vi "Phsae_shift_test(4).vi"() -> ()   [LabVIEW 2017]
uses:
  <vilib>/Analysis/3filter.llb/Filter Passband Type.ctl
  <vilib>/Analysis/3filter.llb/FIR Windowed Filter (DBL).vi
  <vilib>/Analysis/NI_AALBase.lvlib
  <vilib>/Analysis/NI_AALPro.lvlib
panel:
  out "S3 signal":waveform(dbl)(graph)
  out "S2 signal":waveform(dbl)(graph)
  out "S1 signal":waveform(dbl)(graph)
  out "S0 signal":waveform(dbl)(graph)
  out "doppler frequency %":dbl
  in  "Carrier Dopphler On":bool
  in  "DpF":dbl=10000.0
  in  "signal Dopphler On":bool
  out "S0 signal(LPF)":waveform(dbl)(graph)
  out "S1 signal(LPF)":waveform(dbl)(graph)
  out "S2 signal(LPF)":waveform(dbl)(graph)
  out "S3 signal(LPF)":waveform(dbl)(graph)
  out "SUM signal":waveform(dbl)(graph)
  out "최대값":dbl
  in  "Delay time.A.1(sec)":dbl=0.5
  in  "Sampling frequency(Hz)":dbl=3000000.0
  in  "Pulse length(sec)":dbl=0.5
  in  "Amplitude(Vpeak)":dbl=1.0
  in  "Frequency(Hz)":dbl=614000.0
  in  "Carrier Frequency(Hz)":dbl=574000.0
  in  "S0 Phsae":dbl=90.0
  in  "S1 Phsae":dbl=-90.0
  in  "S2 Phsae":dbl=-180.0
  in  "S3 Phsae":dbl=-270.0
  in  "S0 Carrier Phsae":dbl=90.0
  in  "S1 Carrier Phsae":dbl=-90.0
  in  "S2 Carrier Phsae":dbl=-180.0
  in  "S3 Carrier Phsae":dbl=-270.0
  out "S0 FFT":waveform(dbl)(graph)
  out "S1 FFT":waveform(dbl)(graph)
  out "S2 FFT":waveform(dbl)(graph)
  out "S3 FFT":waveform(dbl)(graph)
  out "크기":i32
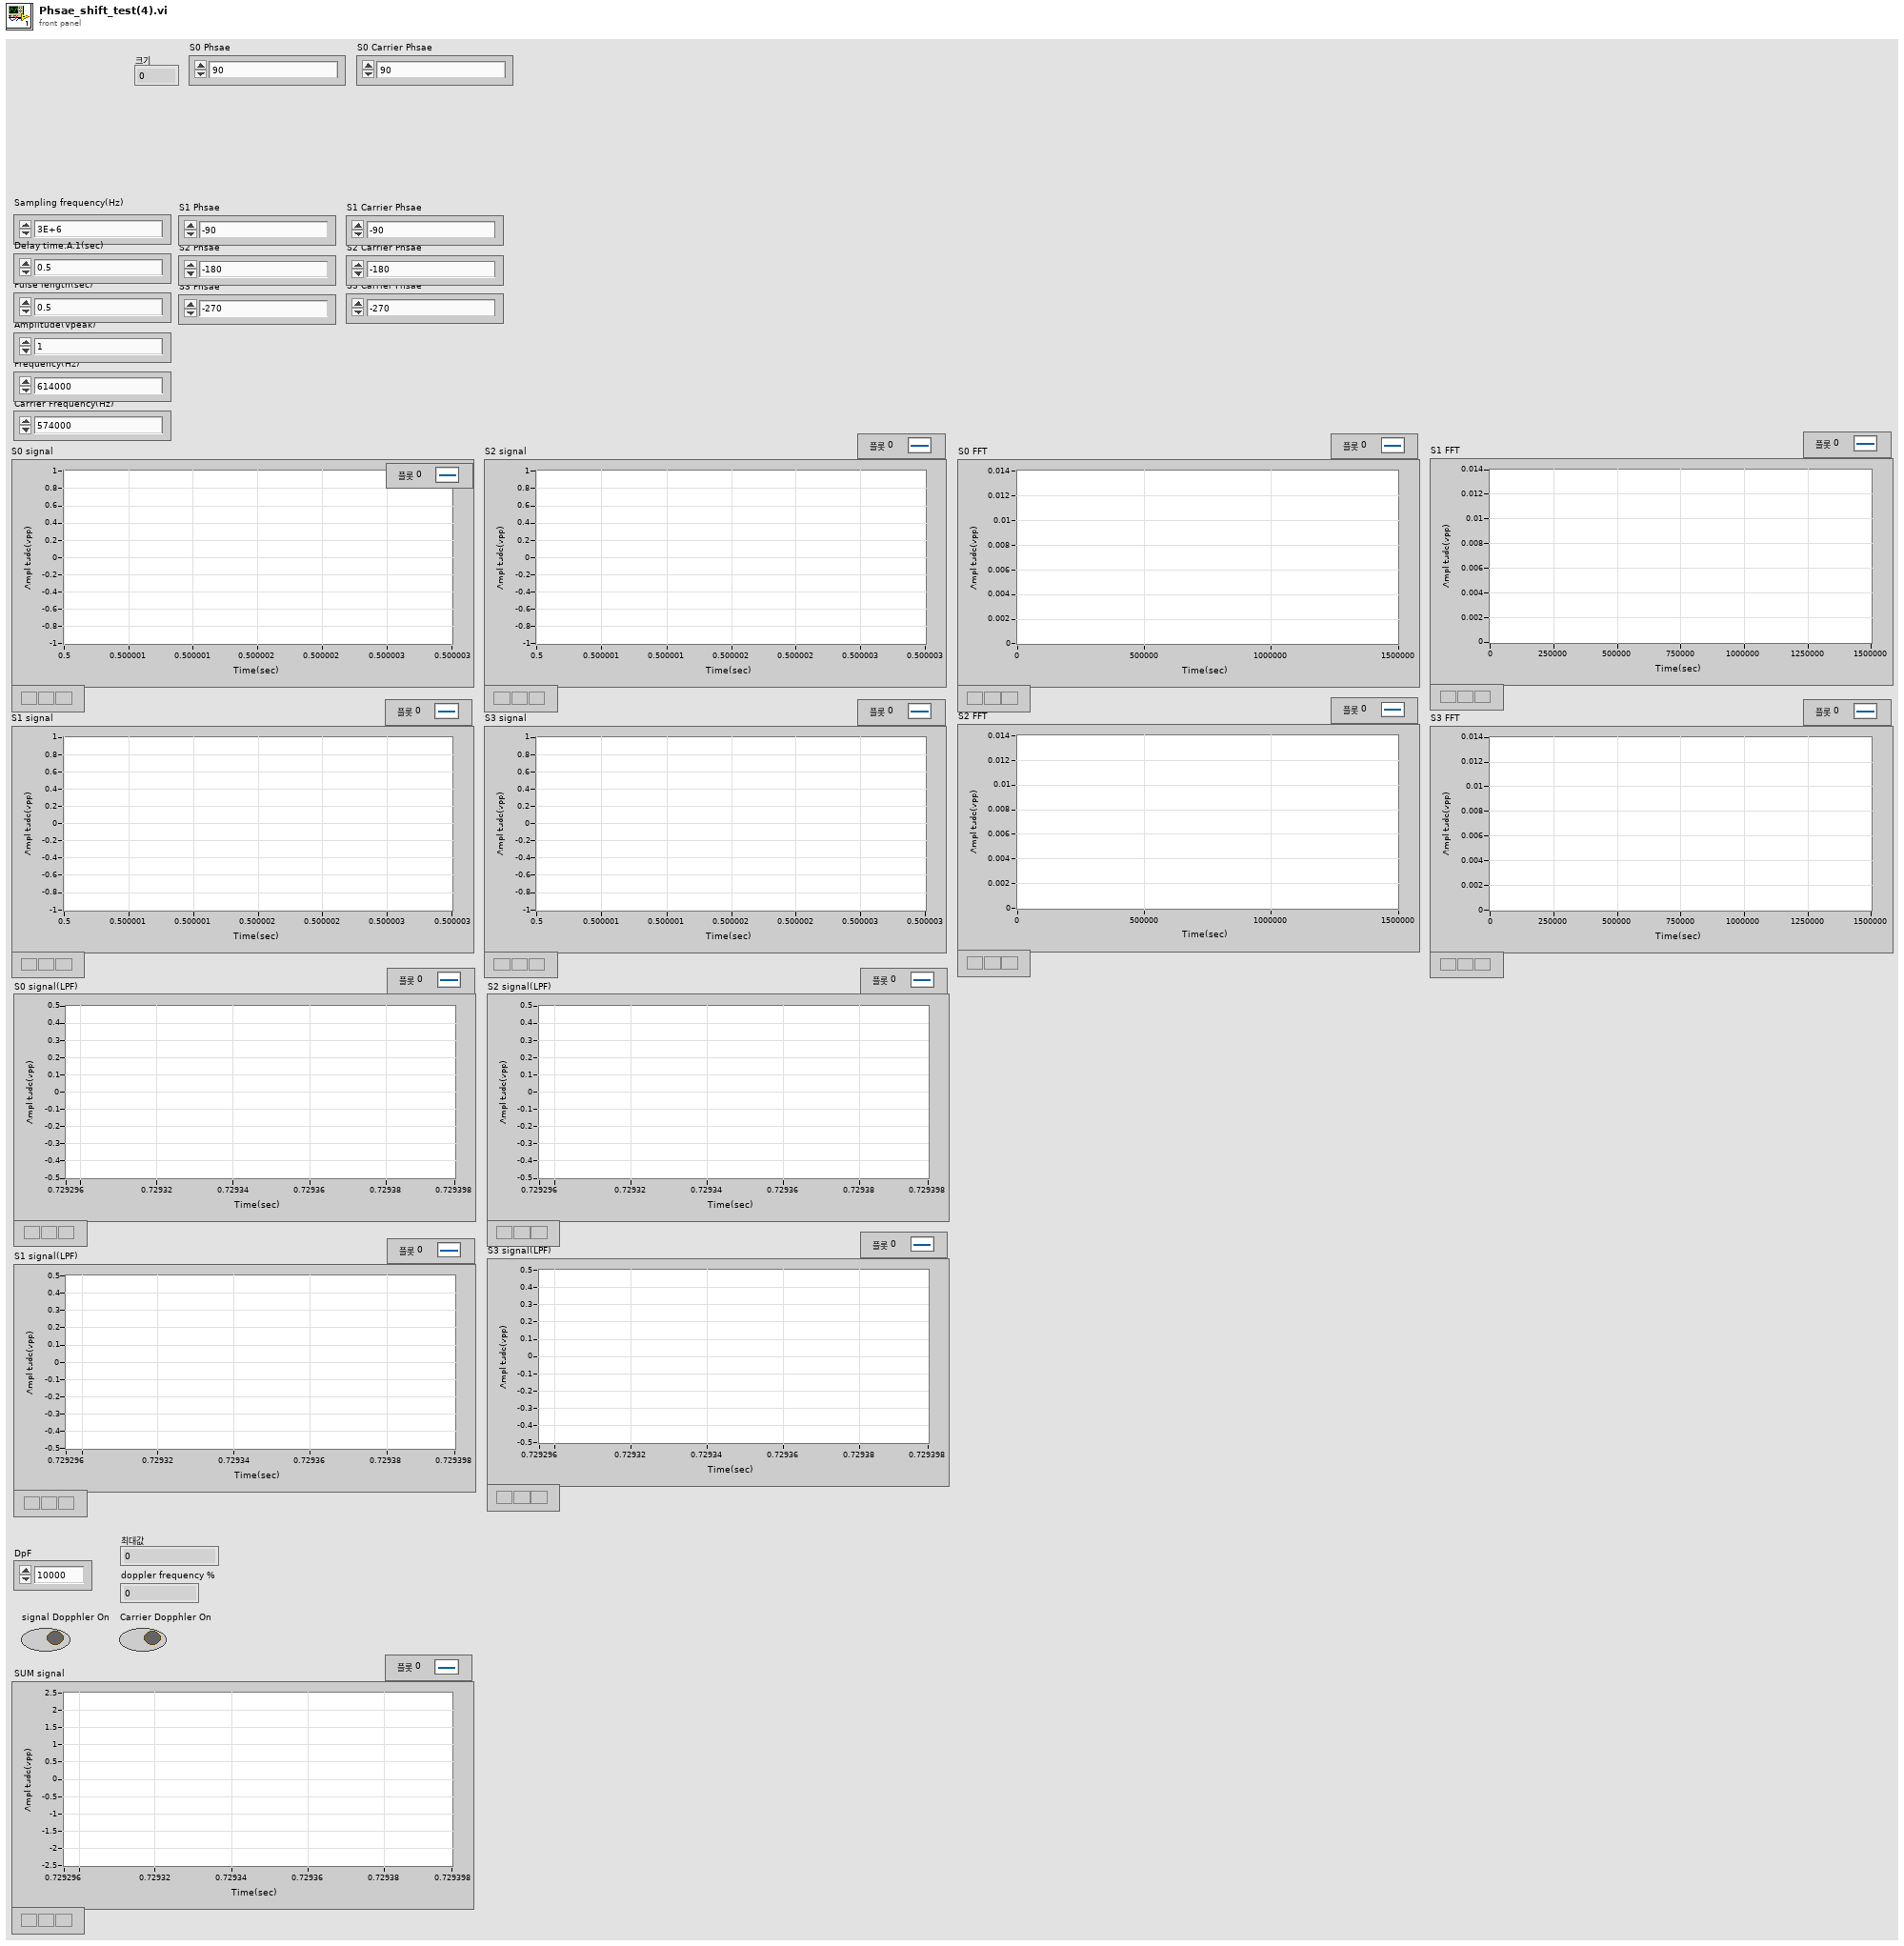
[diagram p1: front panel]
types:
  T1 = typedef "NI_AALBase.lvlib/Filter Passband Type.ctl" = enum32{"Lowpass", "Highpass", "Bandpass", "Bandstop"}
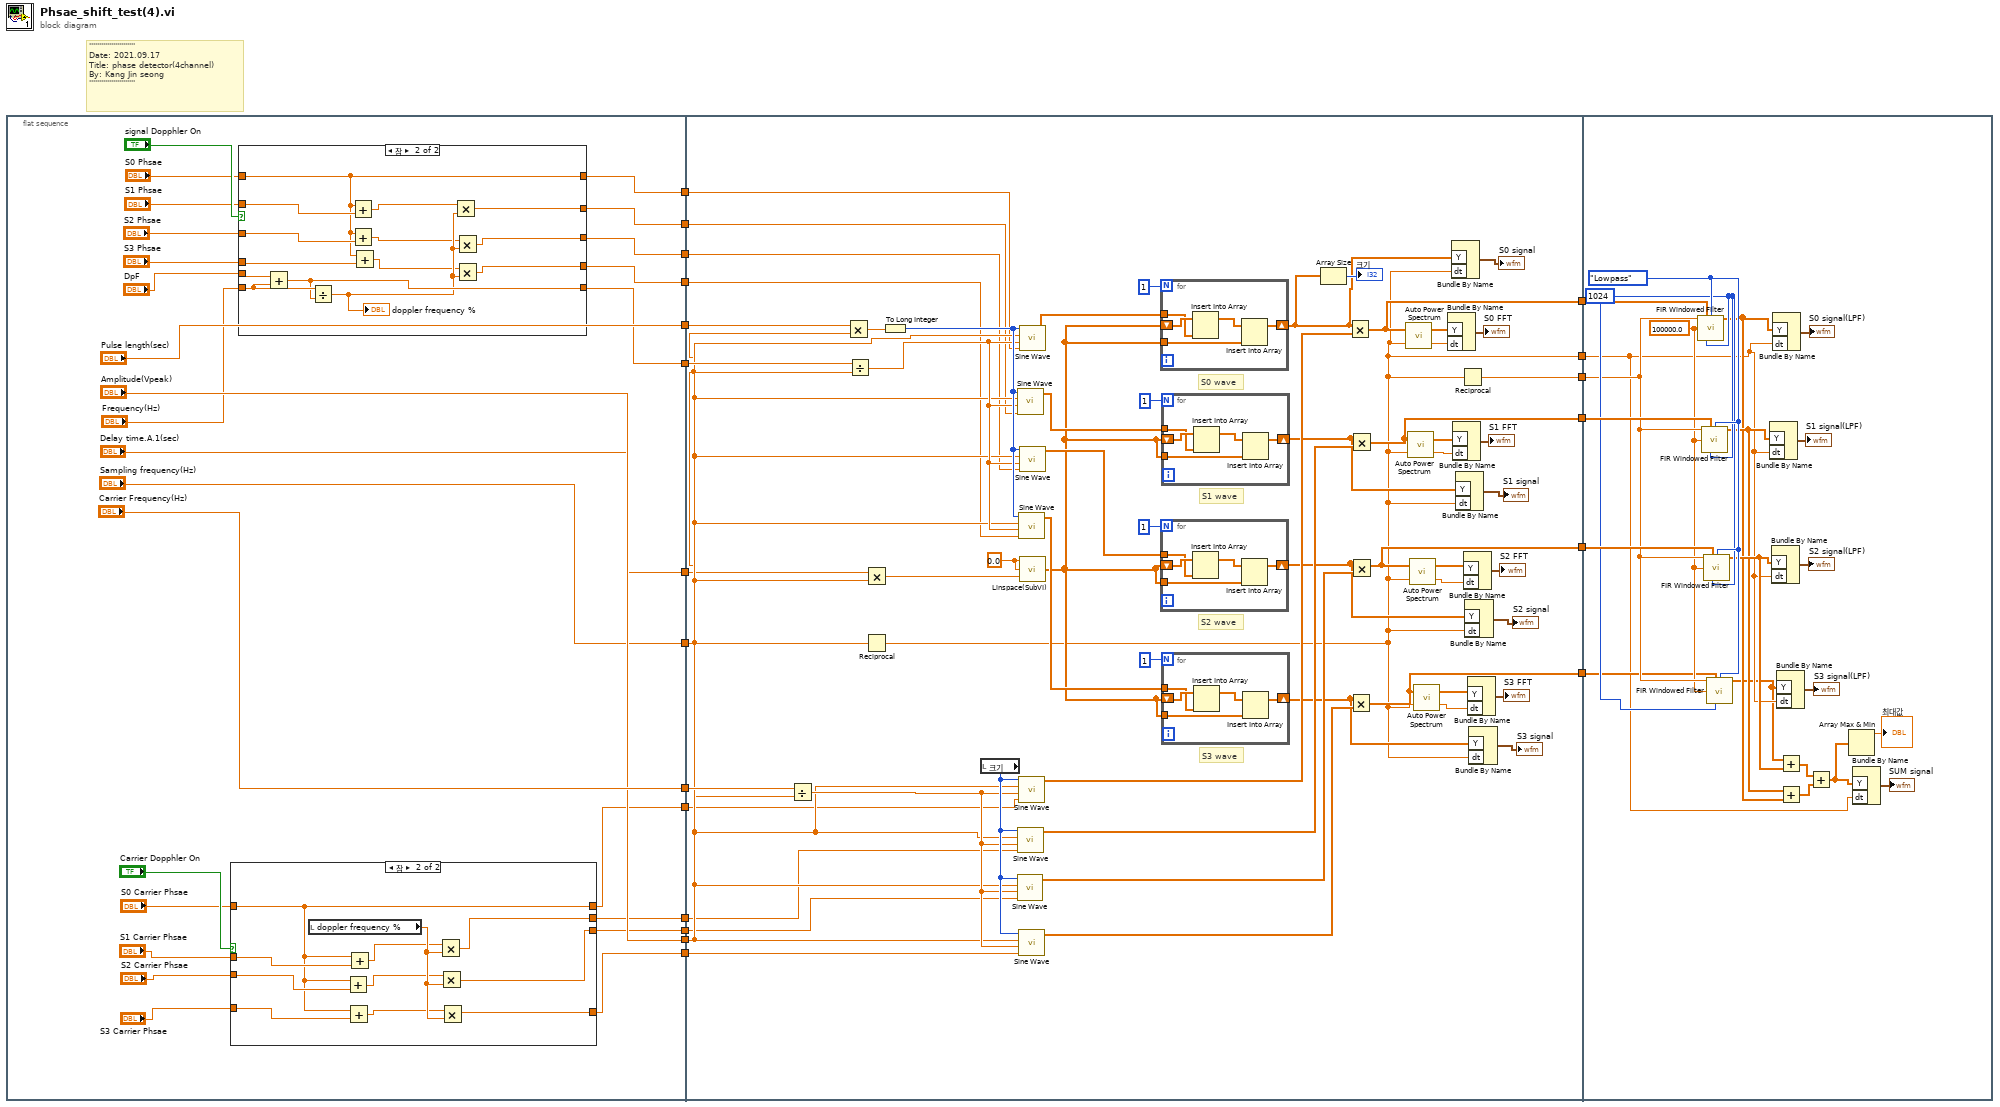
[diagram p0: block diagram]
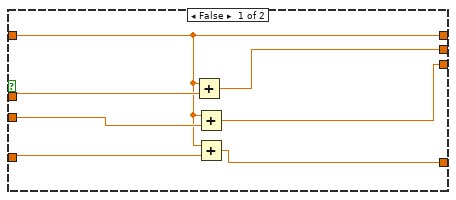
[diagram p2: hidden frame]
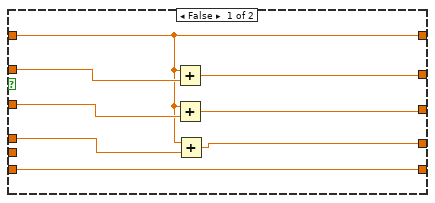
[diagram p3: hidden frame]
diagram:
  # "'''''''''''''''''''''''\nDate: 2021.09.17\nTitle: phase detector(4channel)\nBy: Kang Jin seong\n'''''''''''''''''''''''"
  n1 = flat-sequence {
    tunnel: ["Carrier Frequency(Hz)"] -> w14
    tunnel: [w32] -> w13
    tunnel: ["Amplitude(Vpeak)"] -> w12
    tunnel: ["Pulse length(sec)"] -> w11
    tunnel: ["Sampling frequency(Hz)"] -> w10
    tunnel: ["Delay time.A.1(sec)"] -> w9
    tunnel: [w37] -> w8
    tunnel: [w36] -> w7
    tunnel: [w35] -> w6
    tunnel: [w34] -> w5
    tunnel: [w25] -> w4
    tunnel: [w24] -> w3
    tunnel: [w23] -> w2
    tunnel: [w22] -> w1
    tunnel: [w121] -> w20
    tunnel: [w102] -> w19
    tunnel: [w99] -> w18
    tunnel: [w87] -> w17
    tunnel: [w91] -> w16
    tunnel: [w95] -> w15
    tunnel: w14 -> [w117]
    tunnel: w13 -> [w116]
    tunnel: w12 -> [w115]
    tunnel: w11 -> [w114]
    tunnel: w10 -> [w113]
    tunnel: w9 -> [w112]
    tunnel: w8 -> [w111]
    tunnel: w7 -> [w110]
    tunnel: w6 -> [w109]
    tunnel: w5 -> [w108]
    tunnel: w4 -> [w107]
    tunnel: w3 -> [w106]
    tunnel: w2 -> [w105]
    tunnel: w1 -> [w104]
    tunnel: w15 -> [w182]
    tunnel: w16 -> [w187]
    tunnel: w17 -> [w175]
    tunnel: w18 -> [w188]
    tunnel: w19 -> [w189]
    tunnel: w20 -> [w184]
    frame #0 {
      n2 = case shown="참" "Carrier Dopphler On" {
        tunnel: "S0 Carrier Phsae" -> [w49 w56]
        tunnel: "S1 Carrier Phsae" -> [w53 w60]
        tunnel: "S2 Carrier Phsae" -> [w51 w58]
        tunnel: "S3 Carrier Phsae" -> [w48 w55]
        tunnel: [w49 w56] -> w25
        tunnel: [w52 w63] -> w24
        tunnel: [w50 w62] -> w23
        tunnel: [w47 w61] -> w22
        frame False {
          n3 = Add(x=w49, y=w53) -> (x+y=w52:dbl)
          n4 = Add(x=w49, y=w51) -> (x+y=w50:dbl)
          n5 = Add(x=w49, y=w48) -> (x+y=w47:dbl)
        }
        frame True {
          n6 = local read "doppler frequency %"() -> (w64:dbl)
          n7 = Add(x=w56, y=w58) -> (x+y=w57:dbl)
          n8 = Add(x=w56, y=w55) -> (x+y=w54:dbl)
          n9 = Add(x=w56, y=w60) -> (x+y=w59:dbl)
          n10 = Multiply(x=w59, y=w64) -> (x*y=w63:dbl)
          n11 = Multiply(x=w57, y=w64) -> (x*y=w62:dbl)
          n12 = Multiply(x=w54, y=w64) -> (x*y=w61:dbl)
        }
      }
      n13 = case shown="참" "signal Dopphler On" {
        tunnel: "S0 Phsae" -> [w67 w75]
        tunnel: "S1 Phsae" -> [w71 w79]
        tunnel: "S2 Phsae" -> [w68 w77]
        tunnel: "S3 Phsae" -> [w66 w74]
        tunnel: [w67 w75] -> w37
        tunnel: [w70 w84] -> w36
        tunnel: [w69 w83] -> w35
        tunnel: [w65 w82] -> w34
        tunnel: "Frequency(Hz)" -> [w72 w85]
        tunnel: [w72 w81] -> w32
        tunnel: "DpF" -> [_ w86]
        frame False {
          n14 = Add(x=w67, y=w71) -> (x+y=w70:dbl)
          n15 = Add(x=w67, y=w68) -> (x+y=w69:dbl)
          n16 = Add(x=w67, y=w66) -> (x+y=w65:dbl)
        }
        frame True {
          n17 = Add(x=w86, y=w85) -> (x+y=w81:dbl)
          n18 = Divide(x=w85, y=w81) -> (x/y=w80:dbl)
          "doppler frequency %" <- w80
          n19 = Add(x=w75, y=w79) -> (x+y=w78:dbl)
          n20 = Add(x=w75, y=w77) -> (x+y=w76:dbl)
          n21 = Add(x=w75, y=w74) -> (x+y=w73:dbl)
          n22 = Multiply(x=w78, y=w80) -> (x*y=w84:dbl)
          n23 = Multiply(x=w76, y=w80) -> (x*y=w83:dbl)
          n24 = Multiply(x=w73, y=w80) -> (x*y=w82:dbl)
        }
      }
    }
    frame #1 {
      w144 = 0.0 ("Start")
      # "S3 wave"
      # "S2 wave"
      # "S1 wave"
      # "S0 wave"
      n25 = Divide(x=w117, y=w113) -> (x/y=w132:dbl)
      n26 = Multiply(x=w114, y=w113) -> (x*y=w147:dbl)
      n27 = Divide(x=w116, y=w113) -> (x/y=w145:dbl)
      n28 = Multiply(x=w112, y=w113) -> (x*y=w143:dbl)
      n29 = Reciprocal(x=w113) -> (1/x=w87:dbl)
      n30 = To Long Integer(number=w147) -> (32bit integer=w146:i32)
      n31 = local read "크기"() -> (w133:i32)
      n32 = call <vilib>:"Sine Wave.vi"("samples"=w133, "amplitude"=w115, "frequency"=w132, "phase in"=w105) -> ("sine wave"=w128:dbl[])  [unwired: 1 in, 2 out]
      n33 = call <vilib>:"Sine Wave.vi"("samples"=w146, "amplitude"=w115, "frequency"=w145, "phase in"=w110) -> ("sine wave"=w139:dbl[])  [unwired: 1 in, 2 out]
      n34 = call <vilib>:"Sine Wave.vi"("samples"=w133, "amplitude"=w115, "frequency"=w132, "phase in"=w106) -> ("sine wave"=w129:dbl[])  [unwired: 1 in, 2 out]
      n35 = call <vilib>:"Sine Wave.vi"("samples"=w146, "amplitude"=w115, "frequency"=w145, "phase in"=w108) -> ("sine wave"=w135:dbl[])  [unwired: 1 in, 2 out]
      n36 = call <vilib>:"Sine Wave.vi"("samples"=w133, "amplitude"=w115, "frequency"=w132, "phase in"=w107) -> ("sine wave"=w131:dbl[])  [unwired: 1 in, 2 out]
      n37 = call <vilib>:"Sine Wave.vi"("samples"=w133, "amplitude"=w115, "frequency"=w132, "phase in"=w104) -> ("sine wave"=w127:dbl[])  [unwired: 1 in, 2 out]
      n38 = call <vilib>:"Sine Wave.vi"("samples"=w146, "amplitude"=w115, "frequency"=w145, "phase in"=w111) -> ("sine wave"=w141:dbl[])  [unwired: 1 in, 2 out]
      n39 = call <vilib>:"Sine Wave.vi"("samples"=w146, "amplitude"=w115, "frequency"=w145, "phase in"=w109) -> ("sine wave"=w137:dbl[])  [unwired: 1 in, 2 out]
      n40 = call "Linspace(SubVI).vi"("NumElements"=w143, "End"=w144, "Start"=w144) -> ("Array"=w134:dbl[])
      n41 = for {
        N: 1 -> [_]
        shift-right: [w163] -> w93
        shift-left: w134 -> [w167]
        tunnel: w141 -> [w166]
        tunnel: w134 -> [w164]
        n42 = Insert Into Array(array=w167, new element=w166) -> (w165:dbl[])  [unwired: 1 in]
        n43 = Insert Into Array(array=w165, new element=w164) -> (w163:dbl[])  [unwired: 1 in]
      }
      n44 = for {
        N: 1 -> [_]
        shift-right: [w153] -> w90
        shift-left: w134 -> [w157]
        tunnel: w137 -> [w156]
        tunnel: w134 -> [w154]
        n45 = Insert Into Array(array=w157, new element=w156) -> (w155:dbl[])  [unwired: 1 in]
        n46 = Insert Into Array(array=w155, new element=w154) -> (w153:dbl[])  [unwired: 1 in]
      }
      n47 = for {
        N: 1 -> [_]
        shift-right: [w158] -> w92
        shift-left: w134 -> [w162]
        tunnel: w139 -> [w161]
        tunnel: w134 -> [w159]
        n48 = Insert Into Array(array=w162, new element=w161) -> (w160:dbl[])  [unwired: 1 in]
        n49 = Insert Into Array(array=w160, new element=w159) -> (w158:dbl[])  [unwired: 1 in]
      }
      n50 = for {
        N: 1 -> [_]
        shift-right: [w148] -> w89
        shift-left: w134 -> [w152]
        tunnel: w135 -> [w151]
        tunnel: w134 -> [w149]
        n51 = Insert Into Array(array=w152, new element=w151) -> (w150:dbl[])  [unwired: 1 in]
        n52 = Insert Into Array(array=w150, new element=w149) -> (w148:dbl[])  [unwired: 1 in]
      }
      n53 = Array Size(array=w93) -> (size(s)=→"크기":i32)
      n54 = Multiply(x=w93, y=w131) -> (x*y=w102:dbl[])
      n55 = Multiply(x=w89, y=w127) -> (x*y=w95:dbl[])
      n56 = Multiply(x=w92, y=w129) -> (x*y=w99:dbl[])
      n57 = Multiply(x=w90, y=w128) -> (x*y=w91:dbl[])
      n58 = call <vilib>:"Auto Power Spectrum.vi"("dt"=w87, "Signal (V)"=w102) -> ("df"=w103:dbl, "Power Spectrum (V^2 rms)"=w123:dbl[])
      n59 = call <vilib>:"Auto Power Spectrum.vi"("dt"=w87, "Signal (V)"=w99) -> ("df"=w88:dbl, "Power Spectrum (V^2 rms)"=w122:dbl[])
      n60 = call <vilib>:"Auto Power Spectrum.vi"("dt"=w87, "Signal (V)"=w91) -> ("df"=w97:dbl, "Power Spectrum (V^2 rms)"=w120:dbl[])
      n61 = call <vilib>:"Auto Power Spectrum.vi"("dt"=w87, "Signal (V)"=w95) -> ("df"=w94:dbl, "Power Spectrum (V^2 rms)"=w119:dbl[])
      n62 = Bundle By Name("Y"=w123, "dt"=w103) -> (→"S0 FFT":waveform(dbl))  [unwired: 1 in]
      n63 = Bundle By Name("Y"=w93, "dt"=w87) -> (→"S0 signal":waveform(dbl))  [unwired: 1 in]
      n64 = Bundle By Name("Y"=w122, "dt"=w88) -> (→"S1 FFT":waveform(dbl))  [unwired: 1 in]
      n65 = Bundle By Name("Y"=w92, "dt"=w87) -> (→"S1 signal":waveform(dbl))  [unwired: 1 in]
      n66 = Reciprocal(x=w87) -> (1/x=w121:dbl)
      n67 = Bundle By Name("Y"=w120, "dt"=w97) -> (→"S2 FFT":waveform(dbl))  [unwired: 1 in]
      n68 = Bundle By Name("Y"=w90, "dt"=w87) -> (→"S2 signal":waveform(dbl))  [unwired: 1 in]
      n69 = Bundle By Name("Y"=w119, "dt"=w94) -> (→"S3 FFT":waveform(dbl))  [unwired: 1 in]
      n70 = Bundle By Name("Y"=w89, "dt"=w87) -> (→"S3 signal":waveform(dbl))  [unwired: 1 in]
    }
    frame #2 {
      w186 = Filter_Passband_Type."Lowpass" ("filter type")
      w185 = 1024 ("taps")
      w183 = 100000.0 ("low cutoff freq: fl")
      n71 = call-poly <vilib>:"FIR Windowed Filter.vi"("sampling freq: fs"=w184, "X"=w189, "filter type"=w186, "low cutoff freq: fl"=w183, "taps"=w185) -> ("Filtered X"=w179:dbl[])  [unwired: 9 in, 1 out]
      n72 = call-poly <vilib>:"FIR Windowed Filter.vi"("sampling freq: fs"=w184, "X"=w188, "filter type"=w186, "low cutoff freq: fl"=w183, "taps"=w185) -> ("Filtered X"=w180:dbl[])  [unwired: 9 in, 1 out]
      n73 = call-poly <vilib>:"FIR Windowed Filter.vi"("sampling freq: fs"=w184, "X"=w187, "filter type"=w186, "low cutoff freq: fl"=w183, "taps"=w185) -> ("Filtered X"=w181:dbl[])  [unwired: 9 in, 1 out]
      n74 = call-poly <vilib>:"FIR Windowed Filter.vi"("sampling freq: fs"=w184, "X"=w182, "filter type"=w186, "low cutoff freq: fl"=w183, "taps"=w185) -> ("Filtered X"=w170:dbl[])  [unwired: 9 in, 1 out]
      n75 = Bundle By Name("Y"=w180, "dt"=w175) -> (→"S1 signal(LPF)":waveform(dbl))  [unwired: 1 in]
      n76 = Bundle By Name("Y"=w181, "dt"=w175) -> (→"S2 signal(LPF)":waveform(dbl))  [unwired: 1 in]
      n77 = Bundle By Name("Y"=w179, "dt"=w175) -> (→"S0 signal(LPF)":waveform(dbl))  [unwired: 1 in]
      n78 = Bundle By Name("Y"=w170, "dt"=w175) -> (→"S3 signal(LPF)":waveform(dbl))  [unwired: 1 in]
      n79 = Add(x=w170, y=w181) -> (x+y=w178:dbl[])
      n80 = Add(x=w180, y=w179) -> (x+y=w177:dbl[])
      n81 = Add(x=w178, y=w177) -> (x+y=w169:dbl[])
      n82 = Array Max & Min(array=w169) -> (max value=→"최대값":dbl)  [unwired: 3 out]
      n83 = Bundle By Name("Y"=w169, "dt"=w175) -> (→"SUM signal":waveform(dbl))  [unwired: 1 in]
    }
  }
